vi "core_h5_format_dataset_name.vi"(2 "dataset name in":string) -> (7 "dataset name out":string)   [LabVIEW 2015]
uses:
  <userlib>/_OpenG.lib/string/string.llb/To Camel Case (String)__ogtk.vi
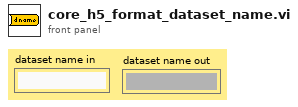
[diagram p1: front panel]
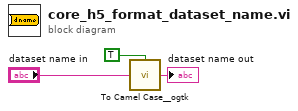
[diagram p0: block diagram]
diagram:
  n1 = call-poly <userlib>:"To Camel Case__ogtk.vi"("string"="dataset name in", "no change if no spaces? (F=No)"=TRUE) -> ("CamelCase string"=→"dataset name out":string)
